vi "cw_6_3.vi"() -> ()   [LabVIEW 2022 SP3]
panel:
  out "Logs 3":string
  out "Logs":string
  out "Logs 2":string
  out "Logs 1":string
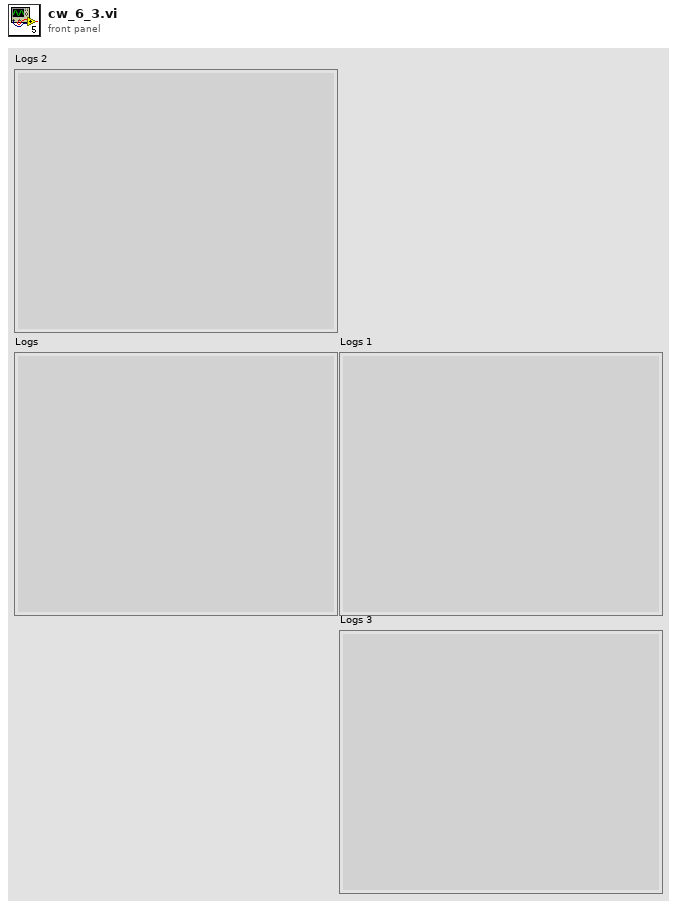
[diagram p1: front panel]
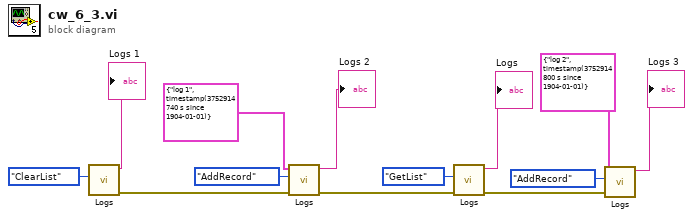
[diagram p0: block diagram]
diagram:
  n1 = call "Logs.vi"("Action"=enum16{"GetList", "AddRecord", "ClearList"}."ClearList") -> ("error out"=w8:errorcluster, "Logs"=→"Logs 1":string)  [unwired: 9 in]
  n2 = call "Logs.vi"("error in"=w8, "Action"=enum16{"GetList", "AddRecord", "ClearList"}."AddRecord", "Cluster"=cluster{"Log":string, "Time Stamp":timestamp} {"Log"="log 1", "Time Stamp"=timestamp(3752914740 s since 1904-01-01)}) -> ("error out"=w7:errorcluster, "Logs"=→"Logs 2":string)  [unwired: 7 in]
  n3 = call "Logs.vi"("error in"=w7, "Action"=enum16{"GetList", "AddRecord", "ClearList"}."GetList") -> ("error out"=w6:errorcluster, "Logs"=→"Logs":string)  [unwired: 8 in]
  n4 = call "Logs.vi"("error in"=w6, "Action"=enum16{"GetList", "AddRecord", "ClearList"}."AddRecord", "Cluster"=cluster{"Log":string, "Time Stamp":timestamp} {"Log"="log 2", "Time Stamp"=timestamp(3752914800 s since 1904-01-01)}) -> ("Logs"=→"Logs 3":string)  [unwired: 7 in, 1 out]
